vi "Proyecto_PuebaDEF_Fuinciona.vi"() -> ()   [LabVIEW 2020]
uses:
  <vilib>/Instr/_visa.llb/VISA Configure Serial Port (Instr).vi
  <vilib>/httpClient/PUTBuffer.vi
  <vilib>/httpClient/LabVIEWHTTPClient.lvlib
panel:
  in  "Tab Control":enum32{"Planta de frijol", "Planta de Maiz"}(tab)
  out "Buen nivel de humedad":bool
  out "Estado Electrovalvula":string
  out "En proceso de regado":bool
  out "Nivel de humedad alto":bool
  in  "Detener mediciones":bool
  out "Indicacion":string
  out "Medio":bool
  out "Lleno":bool
  out "Vacio":bool
  out "Humedad de la planta":dbl(slide) scale=0.0..100.0
  out "Temperactura actual":dbl(slide) scale=0.0..100.0
  out "Estado del suministro":u8(slide)
  out "Estado del suministro":u8(slide)
  out "Temperactura actual":dbl(slide) scale=0.0..100.0
  out "Humedad de la planta":dbl(slide) scale=0.0..100.0
  out "Vacio":bool
  out "Lleno":bool
  out "Medio":bool
  out "Indicacion":string
  in  "Detener mediciones":bool
  out "Buen nivel de hudead":bool
  out "Nivel de humedad alto":bool
  out "En proceso de regado":bool
  out "Estado Electrovalvula":string
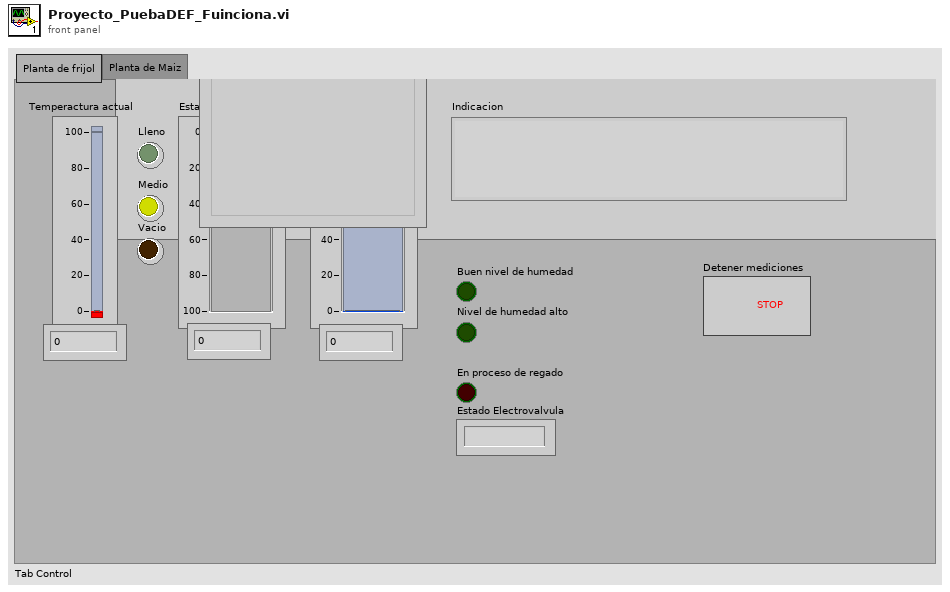
[diagram p1: front panel]
types:
  T1 = cluster{"Fecha":string, "Hora":string, "Humedad":dbl, "Tanque":dbl, "Temperatura":dbl}
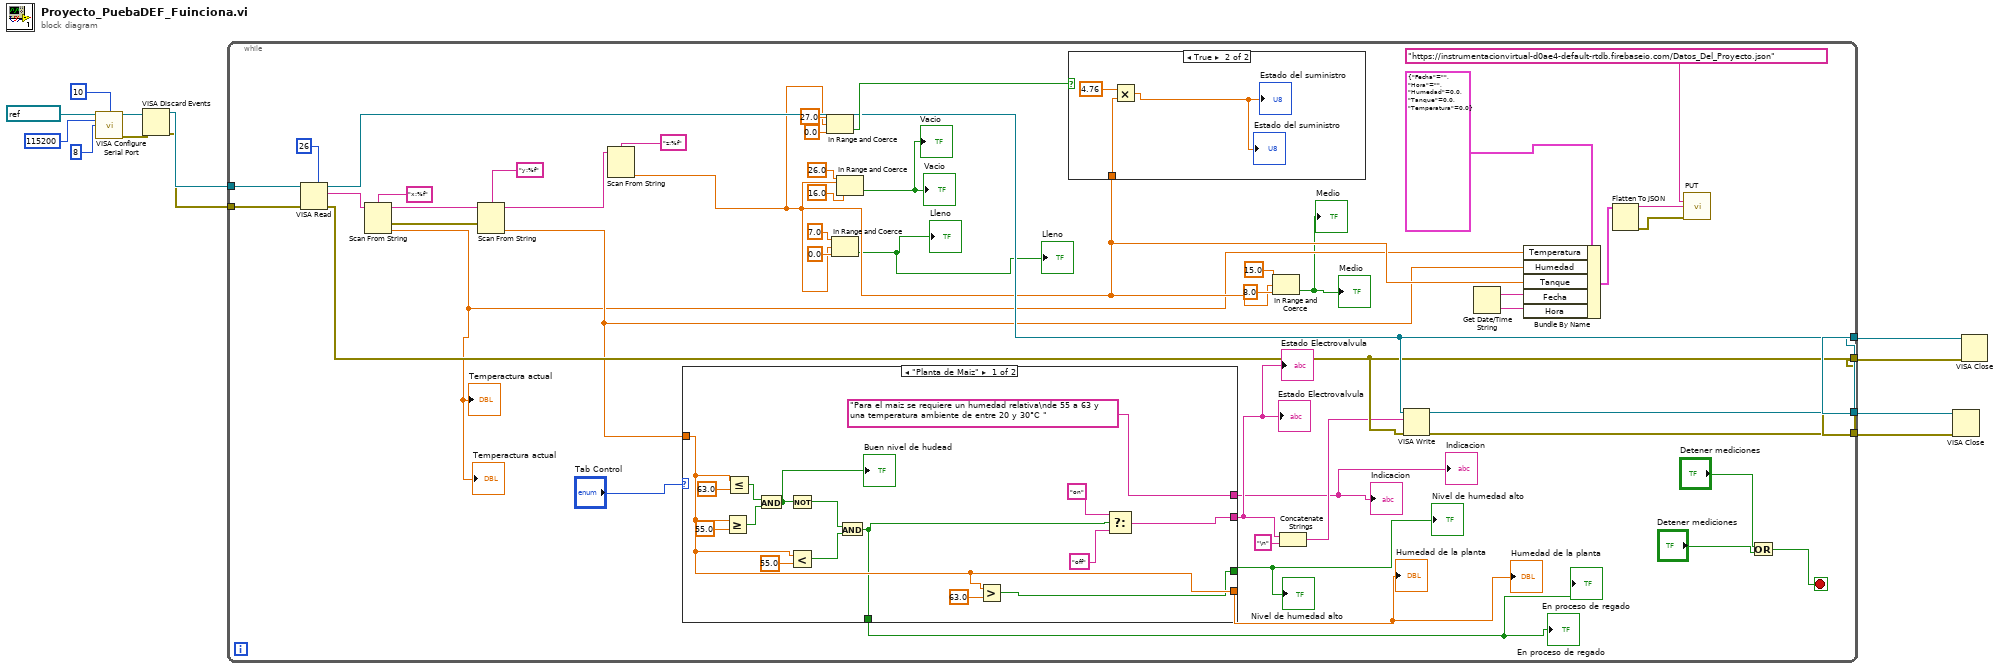
[diagram p0: block diagram]
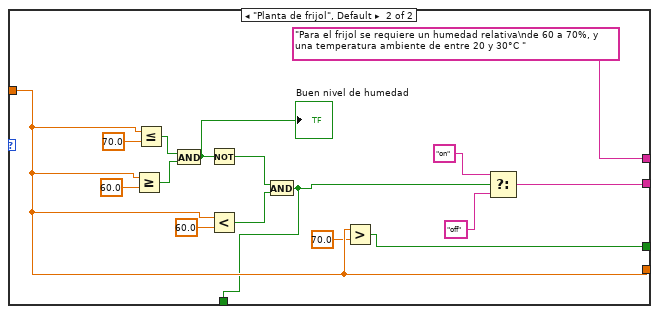
[diagram p2: hidden frame]
diagram:
  n1 = call-poly "VISA Configure Serial Port"("VISA resource name"=refnum<visa-resource-name> "COM6", "termination char\n(0xA = '\\n' = LF)"=u8 10 ("termination char\n(0xA = '\\n' = LF)"), "baud rate (9600)"=u32 115200, "data bits (8)"=u16 8) -> ("VISA resource name out"=w6:refnum<visa-resource-name>, "error out"=w7:errorcluster)  [unwired: 10 in]
  n2 = VISA Discard Events(8:w7, 11:w6) -> (0:w4:errorcluster, 3:w5:refnum<visa-resource-name>)  [unwired: 2 in]
  n3 = while {
    tunnel: [w40] -> w9
    tunnel: [w39] -> w8
    tunnel: w5 -> [w51]
    tunnel: w4 -> [w50]
    tunnel: [w38] -> w2
    tunnel: [w37] -> w1
    stop <- w20 stop-if-true
    n4 = VISA Read(VISA resource name=w51, byte count=u32 26, error in (no error)=w50) -> (VISA resource name out=w40:refnum<visa-resource-name>, read buffer=w57:string, error out=w39:errorcluster)  [unwired: 1 out]
    n5 = Scan From String "Scan From String"(format string="x:%f", input string=w57) -> (remaining string=w56:string, error out=w54:errorcluster, output 1=w19:dbl)  [unwired: 3 in, 1 out]
    "Temperactura actual" <- w19
    "Temperactura actual" <- w19
    n6 = Scan From String "Scan From String"(format string="y:%f", input string=w56, error in=w54) -> (remaining string=w53:string, output 1=w33:dbl)  [unwired: 2 in, 2 out]
    n7 = Scan From String "Scan From String"(format string="z:%f", input string=w53) -> (output 1=w34:dbl)  [unwired: 3 in, 3 out]
    n8 = case shown="\"Planta de Maiz\"" "Tab Control" {
      tunnel: ["Para el maiz se requiere un humedad relativa\nde 55 a 63 y una temperatura ambiente de entre 20 y 30°C " "Para el frijol se requiere un humedad relativa\nde 60 a 70%, y una temperatura ambiente de entre 20 y 30°C "] -> w13
      tunnel: w33 -> [w64 w79]
      tunnel: [w64 w79] -> w23
      tunnel: [w72 w88] -> w14
      tunnel: [w62 w77] -> w24
      tunnel: [w61 w76] -> w15
      frame "Planta de Maiz" {
        n9 = Greater Or Equal?(x=w64, y=55.0) -> (x >= y?=w70:bool)
        n10 = Less Or Equal?(x=w64, y=63.0) -> (x <= y?=w71:bool)
        n11 = And(x=w71, y=w70) -> (x .and. y?=w60:bool)
        "Buen nivel de hudead" <- w60
        n12 = Not(x=w60) -> (.not. x?=w66:bool)
        n13 = Less?(x=w64, y=55.0) -> (x < y?=w67:bool)
        n14 = And(x=w66, y=w67) -> (x .and. y?=w61:bool)
        n15 = Greater?(x=w64, y=63.0) -> (0:w62:bool)
        n16 = Select(t="on", s=w61, f="off") -> (s? t:f=w72:string)
      }
      frame "Planta de frijol", Default {
        n17 = Greater Or Equal?(x=w79, y=60.0) -> (x >= y?=w84:bool)
        n18 = Less Or Equal?(x=w79, y=70.0) -> (x <= y?=w83:bool)
        n19 = And(x=w83, y=w84) -> (x .and. y?=w85:bool)
        "Buen nivel de humedad" <- w85
        n20 = Not(x=w85) -> (.not. x?=w87:bool)
        n21 = Less?(x=w79, y=60.0) -> (x < y?=w86:bool)
        n22 = And(x=w87, y=w86) -> (x .and. y?=w76:bool)
        n23 = Greater?(x=w79, y=70.0) -> (0:w77:bool)
        n24 = Select(t="on", s=w76, f="off") -> (s? t:f=w88:string)
      }
    }
    "Indicacion" <- w13
    "Humedad de la planta" <- w23
    "Nivel de humedad alto" <- w24
    "Estado Electrovalvula" <- w14
    "En proceso de regado" <- w15
    "En proceso de regado" <- w15
    "Nivel de humedad alto" <- w24
    "Humedad de la planta" <- w23
    "Estado Electrovalvula" <- w14
    "Indicacion" <- w13
    n25 = In Range and Coerce(upper limit=27.0, x=w34, lower limit=0.0) -> (In Range?=w49:bool)  [unwired: 1 out]
    n26 = In Range and Coerce(upper limit=7.0, x=w34, lower limit=0.0) -> (In Range?=→"Lleno" →"Lleno":bool)  [unwired: 1 out]
    n27 = In Range and Coerce(upper limit=26.0, x=w34, lower limit=16.0) -> (In Range?=→"Vacio" →"Vacio":bool)  [unwired: 1 out]
    n28 = case shown="True" w49 {
      tunnel: w34 -> [_ w93]
      frame False {
      }
      frame True {
        n29 = Multiply(x=4.76, y=w93) -> (x*y=→"Estado del suministro" →"Estado del suministro":dbl)
      }
    }
    n30 = In Range and Coerce(upper limit=15.0, x=w34, lower limit=8.0) -> (In Range?=→"Medio" →"Medio":bool)  [unwired: 1 out]
    n31 = Concatenate Strings(w14, "\n" ("string")) -> (w26:string)
    n32 = VISA Write(VISA resource name=w40, write buffer=w26, error in (no error)=w39) -> (VISA resource name out=w38:refnum<visa-resource-name>, error out=w37:errorcluster)  [unwired: 1 out]
    n33 = Get Date/Time String() -> (date string=w36:string, time string=w35:string)  [unwired: 3 in]
    n34 = Bundle By Name(cluster=T1 {"Fecha"="", "Hora"="", "Humedad"=0.0, "Tanque"=0.0, "Temperatura"=0.0}, "Temperatura"=w19, "Humedad"=w33, "Tanque"=w34, "Fecha"=w36, "Hora"=w35) -> (w30:T1)
    n35 = Flatten To JSON(anything=w30) -> (JSON string=w31:string, 11:w32:errorcluster)  [unwired: 2 in]
    n36 = call-poly <vilib>:"PUT.vi"("url"="https://instrumentacionvirtual-d0ae4-default-rtdb.firebaseio.com/Datos_Del_Proyecto.json", "buffer"=w31, "error in (no error)"=w32) -> ()  [unwired: 9 in, 4 out]
    n37 = Or(x="Detener mediciones", y="Detener mediciones") -> (x .or. y?=w20:bool)
  }
  n38 = VISA Close(VISA resource name=w9, error in (no error)=w8) -> ()  [unwired: 1 out]
  n39 = VISA Close(VISA resource name=w2, error in (no error)=w1) -> ()  [unwired: 1 out]
